vi "Graph.vi"(8 "error in (no error)":errorcluster, 11 "Collection in":refnum<class "Collection.lvclass">) -> (0 "error out":errorcluster, 2 "Wfm Array":waveform(dbl)[](array[waveform]), 3 "Collection out":refnum<class "Collection.lvclass">)   [LabVIEW 2009, in "Collection.lvclass"]
uses:
  Collection.lvclass
  Collection.lvclass/Collection.ctl
  Readable/Readable.lvclass
panel:
  # "Generate a waveform array for graphing."
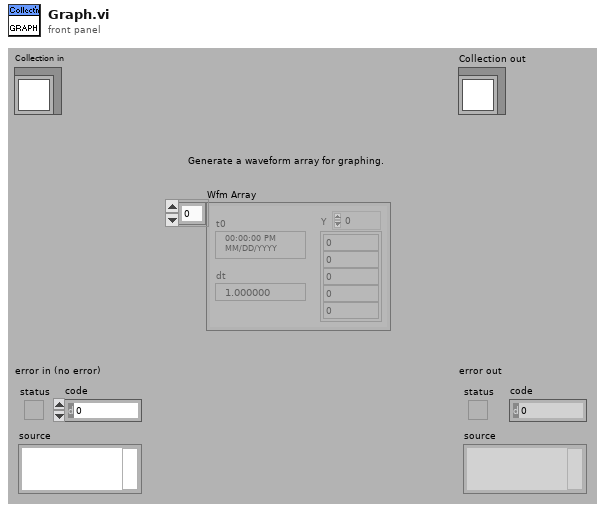
[diagram p1: front panel]
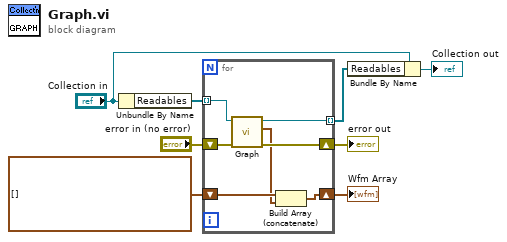
[diagram p0: block diagram]
diagram:
  n1 = Unbundle By Name("Collection in") -> ("Readables"=w8:refnum<class "Readable.lvclass">[])
  n2 = for {
    tunnel: w8 -> [w14] mode=indexing
    shift-right: [w13] -> w5
    shift-left: "error in (no error)" -> [w15]
    shift-right: [w11] -> w6
    shift-left: waveform(dbl)[] [] -> [w10]
    tunnel: [w12] -> w1 mode=indexing
    n3 = call-dynamic "Graph.vi"("error in (no error)"=w15, "Readable in"=w14) -> ("error out"=w13:errorcluster, "Wfm Array"=w9:waveform(dbl)[], "Readable out"=w12:refnum<class "Readable.lvclass">)  [unwired: 7 out]
    n4 = Build Array (concatenate)(w10, w9) -> (w11:waveform(dbl)[])
  }
  "error out" <- w5
  "Wfm Array" <- w6
  n5 = Bundle By Name(cluster="Collection in", "Readables"=w1) -> (→"Collection out":refnum<class "Collection.lvclass">)
